vi "Template delete template from scenario and sequence.vi"(8 "error in (no error)":errorcluster, 10 "deleted template name":string, 11 "Connection Refnum":T1) -> (0 "error out":errorcluster, 3 "Connection Refnum":T1)   [LabVIEW 2011]
uses:
  SI.LIB/ODBC/SQL Controls/Connection Refnum.ctl
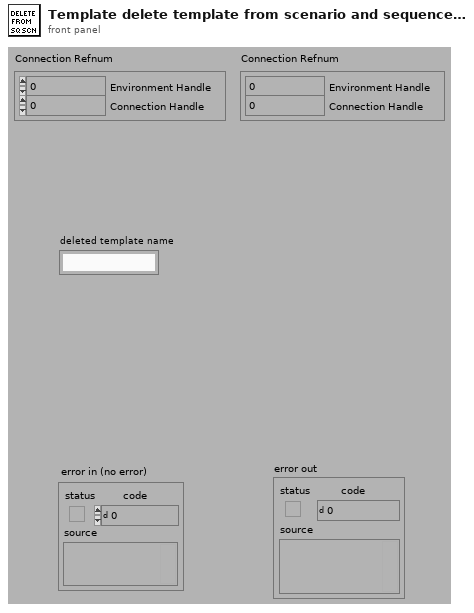
[diagram p1: front panel]
types:
  T1 = typedef "Connection Refnum.ctl" = cluster{"Environment Handle":i32, "Connection Handle":i32}
  T2 = typedef "Scenario Record.ctl" = cluster{"ixScenario":i32, "tCreated":timestamp, "tModified":timestamp, "sxUsername":string, "sModifiedBy":string, "sxScenarioId":string, "sDescription":string, "sLogic":string, "sResultFieldsCSV":string, "sTemplatesCSV":string, "fAutoRunReports":bool, "fSortByTemplates":bool, "fCombinePDF":bool, "Conditions":T3[]}
  T3 = typedef "Condition Record.ctl" = cluster{"iConditionIndex":i32, "sxFieldId":string, "nOperator":T4, "sMatchValue":string}
  T4 = typedef "Condition Operators.ctl" = enum16{"equal (=)", "not equal (\\u2260)", "less than (<)", "less than or equal (\\u2264)", "greater than (>)", "greater than or equal (\\u2265)", "contains", "does not contain"}
  T5 = typedef "Step Record.ctl" = cluster{"ixStep":i32, "sxSequenceId":string, "sxTestId":string, "iIndex":i32, "iRepeat":i32, "iQuickMode":i32, "sTag":string, "sDatasheetsCSV":string, "bConfiguration":string}
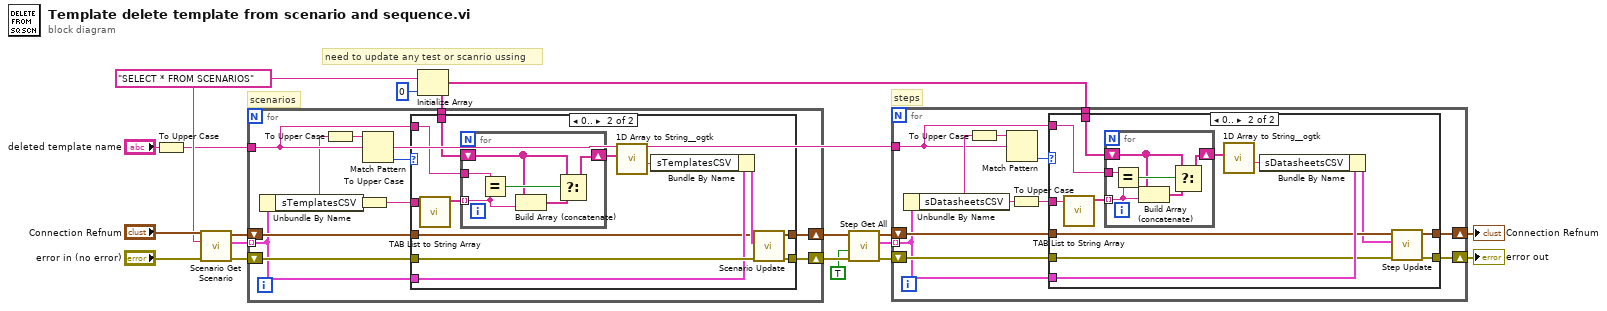
[diagram p0: block diagram]
diagram:
  w14 = "SELECT * FROM SCENARIOS"
  # "steps"
  # "scenarios"
  # "need to update any test or scanrio ussing"
  n1 = To Upper Case(1:"deleted template name") -> (0:w9:string)
  n2 = call "Scenario Get Scenario.vi"("error in (no error)"="error in (no error)", "Query"=w14, "Connection Refnum"="Connection Refnum") -> ("error out"=w17:errorcluster, "Scenarios"=w18:T2[], "Connection Refnum"=w16:T1)  [unwired: 6 out]
  n3 = Initialize Array(w14, 0 ("dimension size")) -> (w7:string[])
  n4 = for {
    tunnel: w18 -> [w22] mode=indexing
    shift-right: [w25] -> w4
    shift-left: w17 -> [w26]
    shift-right: [w23] -> w5
    shift-left: w16 -> [w24]
    tunnel: w9 -> [w21]
    tunnel: w7 -> [w20]
    n5 = Unbundle By Name(w22) -> ("sTemplatesCSV"=w29:string)
    n6 = To Upper Case(1:w29) -> (0:w28:string)
    n7 = To Upper Case(1:w29) -> (0:w19:string)
    n8 = Match Pattern(string=w28, regular expression=w21) -> (offset past match=w27:i32)  [unwired: 4 out]
    n9 = case shown="0.." w27 {
      tunnel: w19 -> [_ w43]
      tunnel: w26 -> [w31 w42]
      tunnel: [w31 w41] -> w25
      tunnel: w24 -> [w30 w37]
      tunnel: [w30 w40] -> w23
      tunnel: w22 -> [_ w39]
      tunnel: w21 -> [_ w35]
      tunnel: w20 -> [_ w34]
      frame Default {
        # "not present"
      }
      frame 0.. {
        n10 = call "TAB List to String Array.vi"("String"=w43) -> ("Array"=w36:string[])  [unwired: 10 out]
        n11 = for {
          tunnel: w36 -> [w44] mode=indexing
          tunnel: w35 -> [w48]
          shift-right: [w47] -> w33
          shift-left: w34 -> [w45]
          n12 = Equal?(x=w48, y=w44) -> (x = y?=w49:bool)
          n13 = Build Array (concatenate)(w45, w44) -> (w46:string[])
          n14 = Select(t=w45, s=w49, f=w46) -> (s? t:f=w47:string[])
        }
        n15 = call "1D Array to String__ogtk.vi"("Array of Strings"=w33) -> ("delimited string"=w32:string)  [unwired: 10 in]
        n16 = Bundle By Name(cluster=w39, "sTemplatesCSV"=w32) -> (w38:T2)
        n17 = call "Scenario Update.vi"("error in (no error)"=w42, "Scenario (none)"=w38, "Connection Refnum"=w37) -> ("error out"=w41:errorcluster, "Connection Refnum"=w40:T1)  [unwired: 7 out]
      }
    }
  }
  n18 = call "Step Get All.vi"("error in (no error)"=w4, "All Steps? (f)"=TRUE, "Connection Refnum"=w5) -> ("error out"=w8:errorcluster, "Sequence Steps"=w11:T5[], "Connection Refnum"=w12:T1)  [unwired: 1 in, 5 out]
  n19 = for {
    shift-right: [w56] -> w2
    shift-left: w8 -> [w57]
    shift-right: [w54] -> w3
    shift-left: w12 -> [w55]
    tunnel: w9 -> [w53]
    tunnel: w11 -> [w50] mode=indexing
    tunnel: w7 -> [w51]
    n20 = Unbundle By Name(w50) -> ("sDatasheetsCSV"=w60:string)
    n21 = To Upper Case(1:w60) -> (0:w59:string)
    n22 = Match Pattern(string=w59, regular expression=w53) -> (offset past match=w58:i32)  [unwired: 4 out]
    n23 = To Upper Case(1:w60) -> (0:w52:string)
    n24 = case shown="0.." w58 {
      tunnel: w52 -> [_ w74]
      tunnel: w57 -> [w62 w67]
      tunnel: [w62 w69] -> w56
      tunnel: w55 -> [w61 w68]
      tunnel: [w61 w70] -> w54
      tunnel: w50 -> [_ w73]
      tunnel: w53 -> [_ w71]
      tunnel: w51 -> [_ w66]
      frame Default {
        # "not present"
      }
      frame 0.. {
        n25 = call "TAB List to String Array.vi"("String"=w74) -> ("Array"=w72:string[])  [unwired: 10 out]
        n26 = for {
          tunnel: w72 -> [w75] mode=indexing
          tunnel: w71 -> [w79]
          shift-right: [w78] -> w64
          shift-left: w66 -> [w76]
          n27 = Equal?(x=w79, y=w75) -> (x = y?=w80:bool)
          n28 = Build Array (concatenate)(w76, w75) -> (w77:string[])
          n29 = Select(t=w76, s=w80, f=w77) -> (s? t:f=w78:string[])
        }
        n30 = call "1D Array to String__ogtk.vi"("Array of Strings"=w64) -> ("delimited string"=w63:string)  [unwired: 10 in]
        n31 = Bundle By Name(cluster=w73, "sDatasheetsCSV"=w63) -> (w65:T5)
        n32 = call "Step Update.vi"("error in (no error)"=w67, "Step Record (empty)"=w65, "Connection Refnum"=w68) -> ("error out"=w69:errorcluster, "Connection Refnum"=w70:T1)  [unwired: 7 out]
      }
    }
  }
  "error out" <- w2
  "Connection Refnum" <- w3
